vi "MEM IO Read Words__ogtk.vi"(4 "error in (no error)":errorcluster, 5 "size":i32 format="%.0x", 6 "type":u16[](array[numeric]), 7 "address":u32 format="%.0x") -> (0 "error out":errorcluster, 2 "data":u16[](array[numeric]))   [LabVIEW 2014]
doc: "This function reads in a number ofwords starting at the specified physical memory adres."
uses:
  <userlib>/_OpenG.lib/portio/ogportio.dll
panel:
  # "[OpenG VI Tags] ***Do Not Remove***"
  # "MEM IO Read Words.vi\n\nReads a number of words from physical memory.\n\nPlease visit http://www.OpenG.org to learn about the\nOpen Source LabVIEW software movement.\n\nNOTICE -- YOU MUST LEAVE THIS NOTICE IN PLACE.  PER THE TERMS OF THE LICENSE BELOW, YOU MAY SUBLICENSE THIS SOFTWARE \nIN ANY WAY THAT DOES NOT CONFLICT WITH THIS LICENSE.\n\n### BSD License (http://www.opensource.org/licenses/bsd-license.php) Begin ###\n\nCopyright (c) 2002-2007, Rolf Kalbermatter <rolf.kalbermatter@citeng.com> \n\nAll rights reserved.\n\nRedistribution and use in source and binary forms, with or without modification, are permitted provided that the following conditions are met:\n\n    * Redistributions of source code must retain the above copyright notice, this list of conditions and the following disclaimer.\n    * Redistributions in binary form must reproduce the above copyright notice, this list of conditions and the following disclaimer in the \n       documentation and/or other materials provided with the distribution.\n    * Neither the name of SciWare, James Kring, Inc., nor the names of its contributors may be used to endorse or promote products derived \n       from this software without specific prior written permission.\n\nTHIS SOFTWARE IS PROVIDED BY THE COPYRIGHT HOLDERS AND CONTRIBUTORS \"AS IS\" AND ANY EXPRESS OR IMPLIED WARRANTIES, \nINCLUDING, BUT NOT LIMITED TO, THE IMPLIED WARRANTIES OF MERCHANTABILITY AND FITNESS FOR A PARTICULAR PURPOSE ARE \nDISCLAIMED. IN NO EVENT SHALL THE COPYRIGHT OWNER OR CONTRIBUTORS BE LIABLE FOR ANY DIRECT, INDIRECT, INCIDENTAL,\n SPECIAL, EXEMPLARY, OR CONSEQUENTIAL DAMAGES (INCLUDING, BUT NOT LIMITED TO, PROCUREMENT OF SUBSTITUTE GOODS OR \nSERVICES; LOSS OF USE, DATA, OR PROFITS; OR BUSINESS INTERRUPTION) HOWEVER CAUSED AND ON ANY THEORY OF LIABILITY, \nWHETHER IN CONTRACT, STRICT LIABILITY, OR TORT (INCLUDING NEGLIGENCE OR OTHERWISE) ARISING IN ANY WAY OUT OF THE USE \nOF THIS SOFTWARE, EVEN IF ADVISED OF THE POSSIBILITY OF SUCH DAMAGE.\n\n### BSD License End ###"
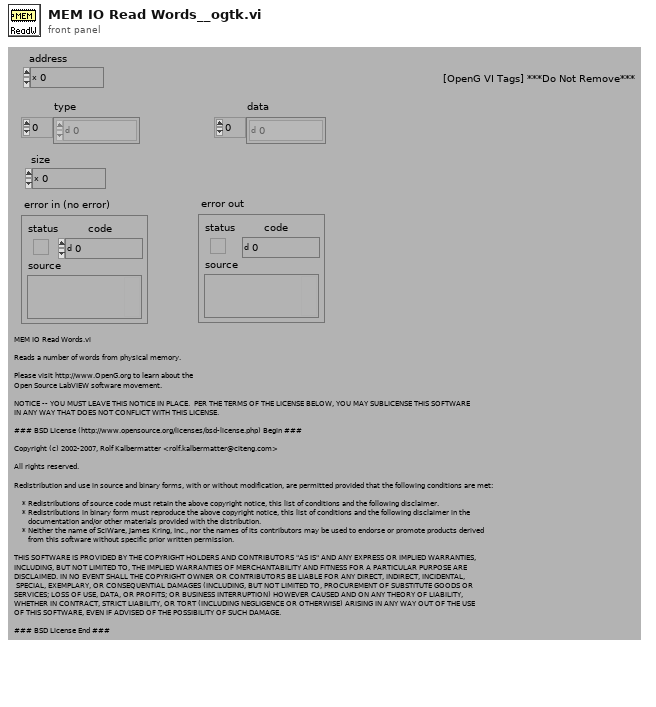
[diagram p1: front panel]
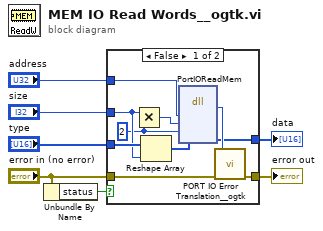
[diagram p0: block diagram]
diagram:
  n1 = Unbundle By Name("error in (no error)") -> ("status"=w7:bool)
  n2 = case shown="False" w7 {
    tunnel: "error in (no error)" -> [w15 w19]
    tunnel: "address" -> [w16 _]
    tunnel: [w14 w19] -> w4
    tunnel: "size" -> [w10 _]
    tunnel: "type" -> [w13 w18]
    tunnel: [w11 w18] -> w1
    frame False {
      w9 = 2 ("unit")
      n3 = Multiply(x=w10, y=w9) -> (x*y=w8:i32)
      n4 = Reshape Array(w13, w10) -> (w12:u16[])
      n5 = dll-call lib="C:/Program Files (x86)/National Instruments/LabVIEW 2014/user.lib/_OpenG.lib/portio/ogportio.*" fn="PortIOReadMem"("address"=w16, "size"=w8, "unit"=w9, "value"=w12) -> (w17:u32, "value"=w11:u16[])  [unwired: 6 in, 2 out]
      n6 = call <userlib>:"PORT IO Error Translation__ogtk.vi"("error in (no error)"=w15, "win error"=w17) -> ("error out"=w14:errorcluster)  [unwired: 5 in]
    }
    frame True {
    }
  }
  "error out" <- w4
  "data" <- w1
